vi "parse string to single end quote.vi"(8 "error in (no error)":errorcluster, 11 "String":string) -> (0 "error out":errorcluster, 3 "string to eol":string)   [LabVIEW 2013]
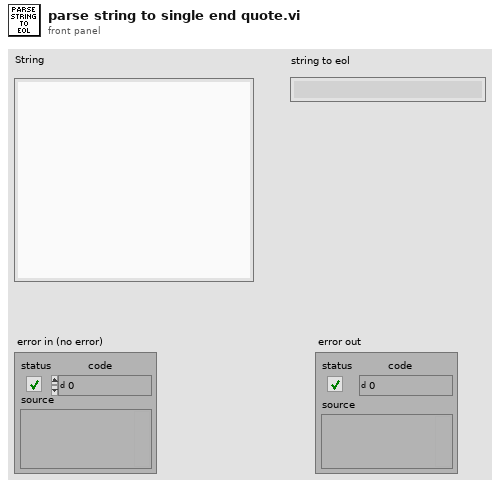
[diagram p1: front panel]
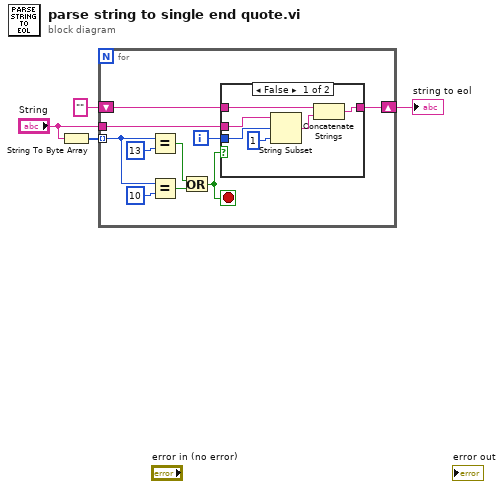
[diagram p0: block diagram]
diagram:
  n1 = String To Byte Array(string="String") -> (unsigned byte array=w4:u8[])
  n2 = for {
    tunnel: w4 -> [w13] mode=indexing
    shift-right: [w6] -> w1
    shift-left: "" -> [w7]
    tunnel: "String" -> [w9]
    i -> [w8]
    stop <- w5 stop-if-true
    n3 = Equal?(x=w13, y=u8 13) -> (x = y?=w11:bool)
    n4 = Equal?(x=w13, y=u8 10) -> (x = y?=w10:bool)
    n5 = Or(x=w11, y=w10) -> (x .or. y?=w5:bool)
    n6 = case shown="False" w5 {
      tunnel: w9 -> [w20 _]
      tunnel: w8 -> [w19 _]
      tunnel: w7 -> [w17 w21]
      tunnel: [w15 w21] -> w6
      frame False {
        n7 = String Subset(string=w20, offset (0)=w19, length (rest)=1 ("length (rest)")) -> (substring=w16:string)
        n8 = Concatenate Strings(w17, w16) -> (w15:string)
      }
      frame True {
      }
    }
  }
  "string to eol" <- w1
